vi "CoerseNumericTypeFixedPoint.vi"(2 "Numeric Variant in":variant, 5 "Numeric":ext) -> (1 "Encoded":string)   [LabVIEW 2021]
uses:
  <vilib>/Utility/Data Type/NI_Data Type.lvlib
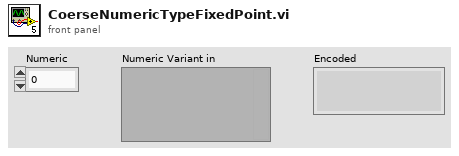
[diagram p1: front panel]
types:
  T1 = typedef "LVFixedPointRepRangeTypeDef.ctl" = cluster{"Range Min":dbl, "Range Max":dbl, "Delta":dbl}
  T2 = typedef "LVFixedPointRepBitsTypeDef.ctl" = cluster{"Signed":bool, "Word Length":u32, "Integer Word Length":i32}
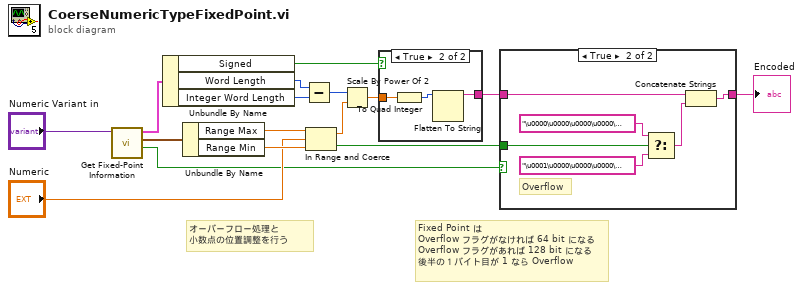
[diagram p0: block diagram]
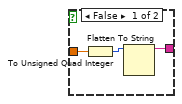
[diagram p3: hidden frame]
diagram:
  # "オーバーフロー処理と\n小数点の位置調整を行う"
  # "Fixed Point は\nOverflow フラグがなければ 64 bit になる\nOverflow フラグがあれば 128 bit になる\n後半の１バイト目が 1 なら Overflow"
  n1 = call <vilib>:"Get Fixed-Point Information.vi"("variant"="Numeric Variant in") -> ("include overflow status?"=w4:bool, "FXP range"=w9:T1, "FXP representation"=w11:T2)  [unwired: 7 in, 1 out]
  n2 = Unbundle By Name(w11) -> ("Signed"=w16:bool, "Word Length"=w12:u32, "Integer Word Length"=w13:i32)
  n3 = Unbundle By Name(w9) -> ("Range Max"=w8:dbl, "Range Min"=w7:dbl)
  n4 = Subtract(x=w12, y=w13) -> (x-y=w14:u32)
  n5 = In Range and Coerce(upper limit=w8, x="Numeric", lower limit=w7) -> (coerced(x)=w5:ext, In Range?=w3:bool)
  n6 = Scale By Power Of 2(n=w14, x=w5) -> (x*2^n=w15:ext)
  n7 = case shown="True" w16 {
    tunnel: w15 -> [w19 w22]
    tunnel: [w17 w20] -> w2
    frame False {
      n8 = To Unsigned Quad Integer(1:w19) -> (0:w18:u64)
      n9 = Flatten To String(anything=w18) -> (data string=w17:string)  [unwired: 3 in, 2 out]
    }
    frame True {
      n10 = To Quad Integer(1:w22) -> (0:w21:i64)
      n11 = Flatten To String(anything=w21) -> (data string=w20:string)  [unwired: 3 in, 2 out]
    }
  }
  n12 = case shown="True" w4 {
    tunnel: w3 -> [_ w28]
    tunnel: w2 -> [w23 w25]
    tunnel: [w23 w24] -> w1
    frame False {
    }
    frame True {
      # "Overflow"
      n13 = Select(t="\u0000\u0000\u0000\u0000\u0000\u0000\u0000\u0000", s=w28, f="\u0001\u0000\u0000\u0000\u0000\u0000\u0000\u0000") -> (s? t:f=w26:string)
      n14 = Concatenate Strings(w25, w26) -> (w24:string)
    }
  }
  "Encoded" <- w1
